vi "Precision.vi"(0 "String":string, 7 "Loop Index":i32, 11 "CmdStep":dbl format="%.5f") -> (8 "Digits of Precision":i32)   [LabVIEW 2019]
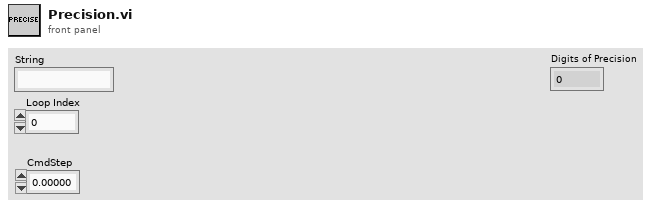
[diagram p1: front panel]
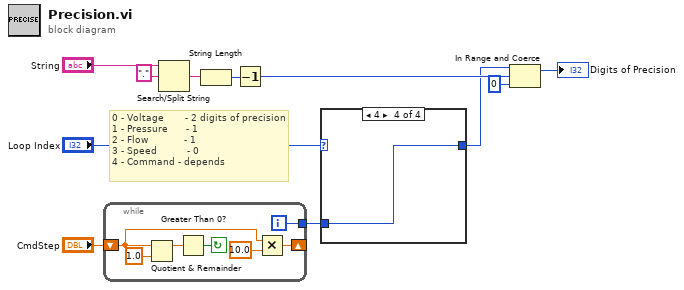
[diagram p0: block diagram]
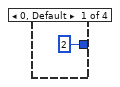
[diagram p2: hidden frame]
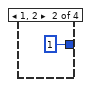
[diagram p3: hidden frame]
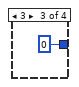
[diagram p4: hidden frame]
diagram:
  # "0 - Voltage       - 2 digits of precision\n1 - Pressure      - 1 \n2 - Flow            - 1\n3 - Speed          - 0\n4 - Command - depends"
  n1 = while {
    shift-right: [w13] -> _
    shift-left: "CmdStep" -> [w12]
    tunnel: [w15] -> w1
    i -> [w15]
    stop <- w16 continue-if-true
    n2 = Quotient & Remainder(x=w12, y=1.0) -> (x-y*floor(x/y)=w17:dbl)  [unwired: 1 out]
    n3 = Greater Than 0?(x=w17) -> (x > 0?=w16:bool)
    n4 = Multiply(x=w12, y=10.0) -> (x*y=w13:dbl)
  }
  n5 = Search/Split String(string="String", search string/char (-)="." ("regular expression")) -> (match + rest of string=w7:string)  [unwired: 1 in, 2 out]
  n6 = String Length(string=w7) -> (length=w8:i32)
  n7 = Decrement(x=w8) -> (x-1=w9:i32)
  n8 = case shown="4" "Loop Index" {
    tunnel: [2 ("Loop Index") 1 ("Loop Index") 0 ("Loop Index") w22] -> w2
    tunnel: w1 -> [_ _ _ w22]
    frame 0, Default {
    }
    frame 1, 2 {
    }
    frame 3 {
    }
    frame 4 {
    }
  }
  n9 = In Range and Coerce(upper limit=w2, x=w9, lower limit=0) -> (coerced(x)=→"Digits of Precision":i32)  [unwired: 1 out]
